vi "Example2_Week5.vi"() -> ()   [LabVIEW 2021, in "LabVIEW Interface for Arduino.lvlib"]
doc: "An example that uses the Arduino to read the value of a photocell."
uses:
  <vilib>/LabVIEW Interface for Arduino/LabVIEW Interface for Arduino.lvlib
  <vilib>/LabVIEW Interface for Arduino/Type Defs/Analog Pin.ctl
panel:
  out "Light Sens":bool
  in  "Digital Pin":dbl
  in  "VISA resource":refnum<visa-resource-name>
  in  "Stop":bool
  out "Light Intensity (0 - 100)":dbl(knob) scale=0.0..100.0
  in  "Photo Cell Pin (AI 0-5)":T1=enum."Anlog In 1"
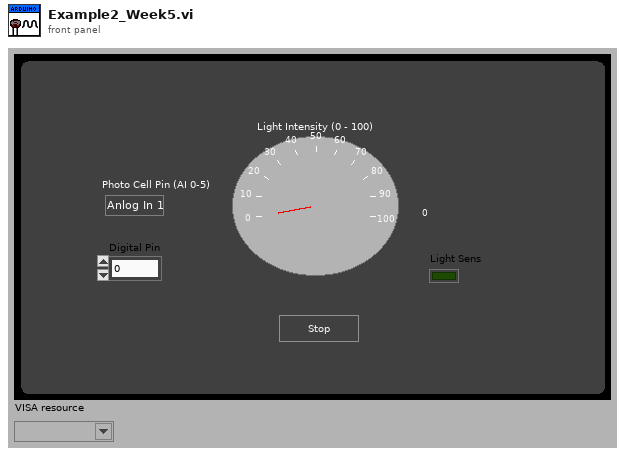
[diagram p1: front panel]
types:
  T1 = typedef "LabVIEW Interface for Arduino.lvlib/Analog Pin.ctl" = enum8{"Anlog In 0", "Anlog In 1", "Anlog In 2", "Anlog In 3", "Anlog In 4", "Anlog In 5"}
  T2 = typedef "LabVIEW Interface for Arduino.lvlib/Arduino Resource.ctl" = cluster{"VISA resource":refnum<visa-resource-name>, "Board Type":T3, "Connection Type":enum8{"USB / Serial"}, "Bytes Per Packet (15)":u8}
  T3 = typedef "LabVIEW Interface for Arduino.lvlib/Board Type.ctl" = enum16{"Uno", "Dimuelanove w/Atmega 328", "Mega 2560"}
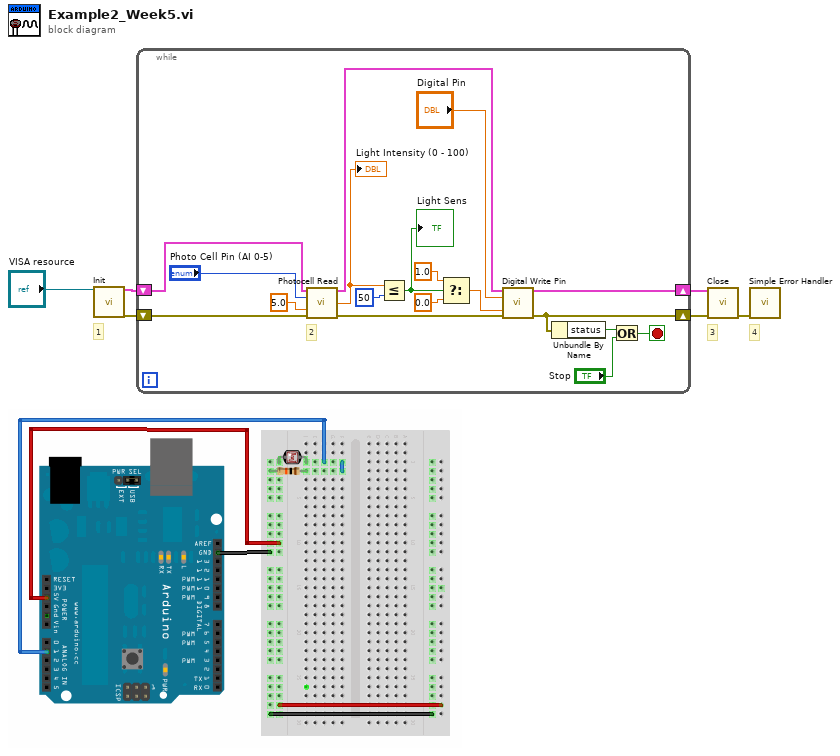
[diagram p0: block diagram]
diagram:
  # "4"
  # "3"
  # "1"
  n1 = call <vilib>:"Init.vi"(0:"VISA resource") -> ("Arduino Resource"=w5:T2, "error out"=w4:errorcluster)  [unwired: 17 in]
  n2 = while {
    shift-right: [w12] -> w6
    shift-left: w4 -> [w24]
    shift-right: [w14] -> w2
    shift-left: w5 -> [w18]
    stop <- w19 stop-if-true
    # "2"
    n3 = call <vilib>:"Photocell Read.vi"("Arduino Resource"=w18, "Photo Cell Pin (0)"="Photo Cell Pin (AI 0-5)", "Vcc (5)"=5.0 ("Vcc"), "error in"=w24) -> ("Arduino Resource"=w15:T2, "Light Intensity (0 - 100)"=w17:dbl, "error out"=w13:errorcluster)  [unwired: 9 in]
    "Light Intensity (0 - 100)" <- w17
    n4 = Less Or Equal?(x=w17, y=50) -> (x <= y?=w7:bool)
    "Light Sens" <- w7
    n5 = Select(t=1.0, s=w7, f=0.0) -> (s? t:f=w8:dbl)
    n6 = call <vilib>:"Digital Write Pin.vi"("Arduino Resource"=w15, "Digital I/O Pin (0)"="Digital Pin", "Value (0)"=w8, "error in"=w13) -> ("Arduino Resource"=w14:T2, "error out"=w12:errorcluster)  [unwired: 10 in]
    n7 = Unbundle By Name(w12) -> ("status"=w21:bool)
    n8 = Or(x=w21, y="Stop") -> (x .or. y?=w19:bool)
  }
  n9 = call <vilib>:"Close.vi"("Arduino Resource"=w2, "error in"=w6) -> ("error out"=w3:errorcluster)  [unwired: 13 in]
  n10 = call <vilib>:"Simple Error Handler.vi"("error in (no error)"=w3) -> ()  [unwired: 4 in, 5 out]
